vi "TCU Module (Main).vi"(7 "Name of Parent Panel":string="Main.vi", 9 "New Center Coords":T1={"Horizontal"=470, "Vertical"=200}, 10 "Config":variant, 11 "Main UI Message Queue":refnum<queue>) -> ()   [LabVIEW 2018, in "TCU Module.lvlib"]
doc: "This Continuous Measurement sample project is based on the Queued Message Handler template.\n\nThe Event Handling Loop generates messages based on user interface actions.\n\nThe Message Handling Loop processes messages generated by the Event Handling Loop, or by other messages. There are also Acquisition and Logging message handling loop subVIs, and a chart updating loop."
uses:
  TCU Module.lvlib
  support/Message Queue/Message Cluster.ctl
  <vilib>/Utility/miscctls.llb/LVPoint32TypeDef.ctl
  controls/UI Data.ctl
  controls/UI State.ctl
  TCU Module State Cluster.ctl
  TCU Module Config Cluster.ctl
  TCU Module Settings Cluster.ctl
  Measure Instrument/Output Devices.ctl
  Huber TCU/Huber Settings.ctl
  Lauda Integral XT-150 TCU/Lauda Settings.ctl
  Julabo Type 1 TCU/Julabo Type 1 TCU Folder/Julabo FP-50 Settings.ctl
  Huber Unistat 410 TCU/Huber Unistat 410 RS485 Settings.ctl
  Measure Instrument/State Enum.ctl
  Sequencing/Squence Update Cluster.ctl
  TCU Module Display.ctl
  support/Message Queue/Enqueue Message (Single).vi
  support/User Event - Stop/User Event - Stop.lvlib
  support/Support Library.lvlib
  support/Message Queue/Message Queue.lvlib
  Measure Instrument/TCU Module Engine.lvlib
  Measure Instrument/Feed Module Engine.lvlib
  Huber TCU/Huber Ministat 230 TCU.lvlib
  Lauda Integral XT-150 TCU/Lauda TCU.lvlib
  Julabo Type 1 TCU/Julabo Type 1 TCU Folder/Julabo Type FP-50 TCU.lvlib
  Sequencing/Sequencing Library.lvlib
  support/Command Log VIs/Command Logging.lvlib
  Huber Unistat 410 TCU/Huber Unistat 410 TCU.lvlib
  Report Generation/Report Generation.lvlib
panel:
  in  "Settings Button":bool
  out "Display Cluster":cluster{"User Name":string, "Temp Display":dbl}
  out "H/W":dbl
  out "Original Height":u32
  out "Original Width":u32
  out "TCU Image":u16(ring)
  out "TCU On?":bool
  out "ScanCode":i16
  out "Log File path":path
  out "Status":string
  in  "Exit":bool
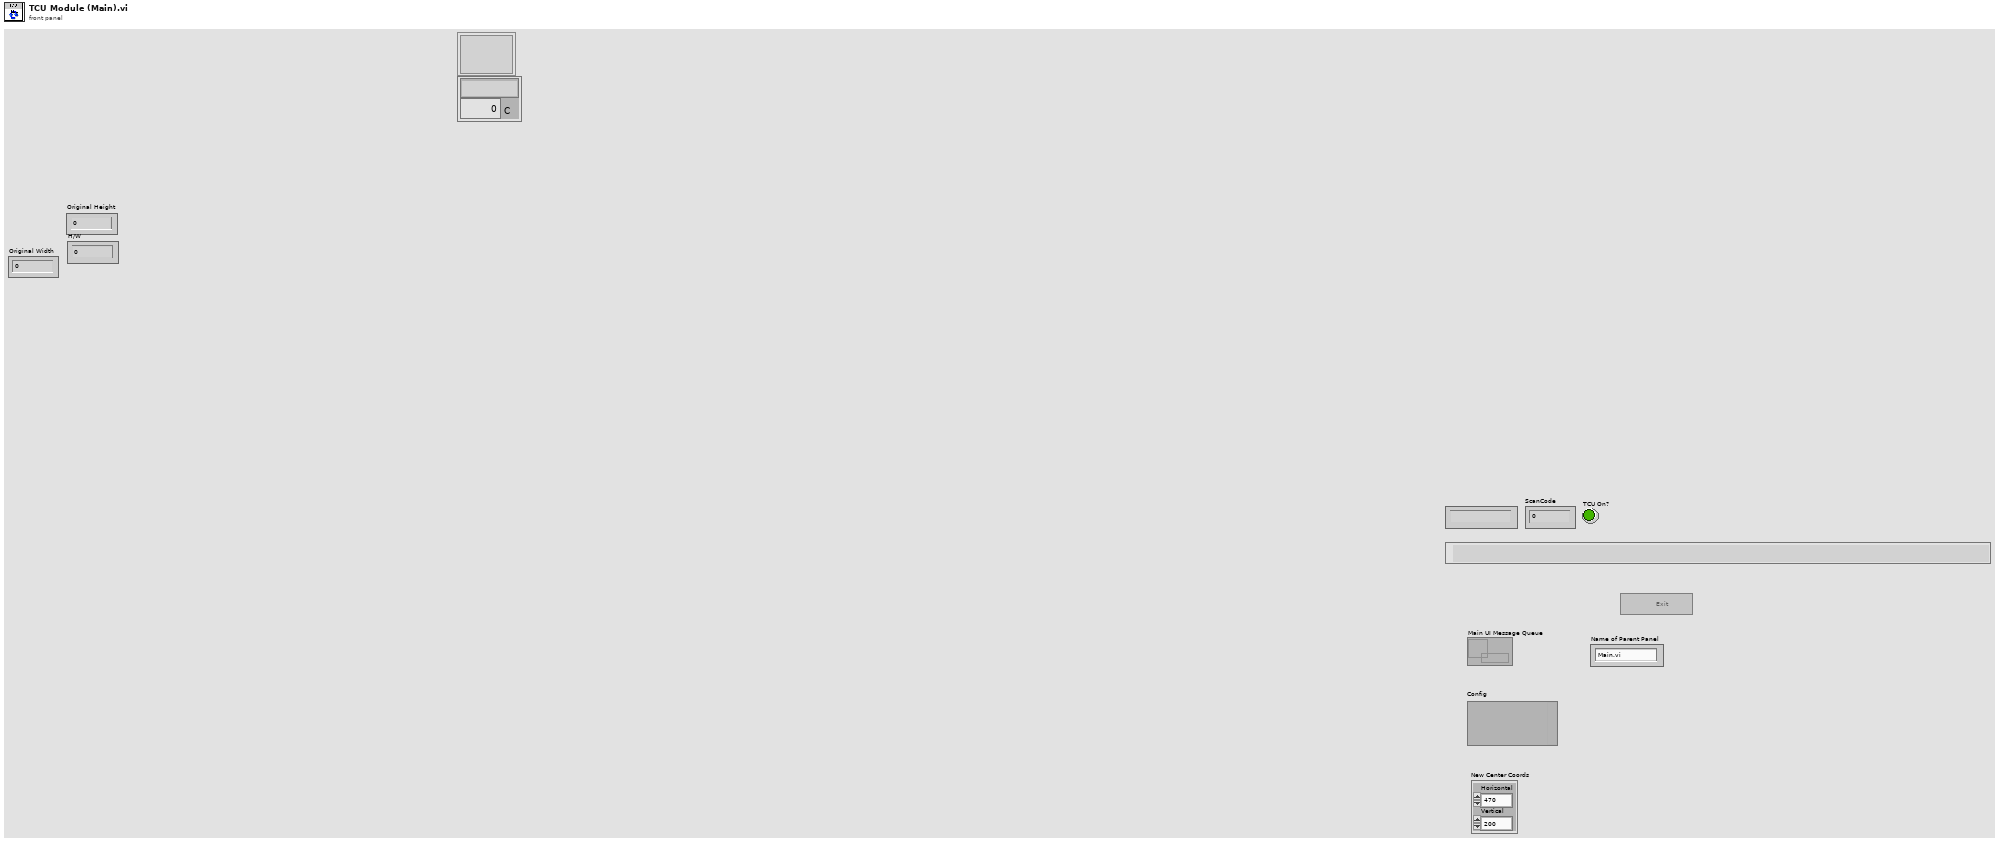
[diagram p1: front panel]
types:
  T1 = typedef "LVPoint32TypeDef.ctl" = cluster{"Horizontal":i32, "Vertical":i32}
  T2 = enum32{"Invalid", "Default", "Floating", "Floating/Auto-Hide", "Modal"}
  T3 = typedef "UI State.ctl" = enum16{"Idle", "Acquiring and Logging", "Waiting for Exit", "Waiting for Exit (Acq Stopped)", "Waiting for Exit (Log Stopped)", "Waiting for Stop", "Waiting for Stop (Acq Stopped)", "Waiting for Stop (Log Stopped)"}
  T4 = typedef "UI Data.ctl" = cluster{"Start Ref":refnum<vi>, "Trigger Ref":refnum<vi>, "Stop Ref":refnum<vi>, "Settings Ref":refnum<vi>, "Status Ref":refnum<vi>, "Exit Ref":refnum<vi>, "Data Ref":refnum<vi>}
  T5 = typedef "TCU Module.lvlib/TCU Module Config Cluster.ctl" = cluster{"GUID":string, "Drop Coords":T1, "Process Name":string, "User name":string, "Queue Name":string, "Settings":T6, "Load Count":i32, "Power Level Changed":bool}
  T6 = typedef "TCU Module.lvlib/TCU Module Settings Cluster.ctl" = cluster{"Cycle Period":dbl, "Setpoint Entry":dbl, "Output Device":T7, "Huber Ministat 230 Settings":T8, "Lauda Settings":T9, "Julabo FP-50 Settings":T10, "Internal Control?":bool, "Huber Unistat 410 Settings":T11}
  T7 = typedef "Output Devices.ctl" = enum16{"Default", "Huber Ministat 230", "Huber Unistat 410", "Lauda XT-150", "Julabo FP-50"}
  T8 = typedef "Huber Ministat 230 TCU.lvlib/Huber Settings.ctl" = cluster{"VISA resource name":refnum<visa-resource-name>, "Simulated?":bool}
  T9 = typedef "Lauda TCU.lvlib/Lauda Settings.ctl" = cluster{"VISA resource name":refnum<visa-resource-name>, "Simulated?":bool, "Pump Power":i32}
  T10 = typedef "Julabo Type FP-50 TCU.lvlib/Julabo FP-50 Settings.ctl" = cluster{"VISA resource name":refnum<visa-resource-name>, "Simulated?":bool, "Pump Power":i32}
  T11 = typedef "Huber Unistat 410 TCU.lvlib/Huber Unistat 410 RS485 Settings.ctl" = cluster{"VISA resource name":refnum<visa-resource-name>, "Address":i8, "Simulated?":bool}
  T12 = typedef "TCU Module.lvlib/TCU Module State Cluster.ctl" = cluster{"TCU Module Config":T5, "State":T13, "Start Time":timestamp, "Current Time":timestamp, "First Iteration":bool, "Data":cluster{"TCU Temp":dbl}, "Process Name":string, "TCU On?":bool, "Power Level Changed":bool}
  T13 = typedef "Feed Module.lvlib/Feed Module Engine.lvlib/State Enum.ctl" = enum16{"Measuring", "Idle", "Paused"}
  T14 = typedef "LVPointTypeDef.ctl" = cluster{"Horizontal":i16, "Vertical":i16}
  T15 = typedef "TCU Module.lvlib/All Message Queues.ctl" = cluster{"Engine":refnum<queue>, "TCU UI":refnum<queue>, "TCU Engine":refnum<queue>, "TCU Display":refnum<queue>}
  T16 = typedef "TCU Module.lvlib/TCU Module Display.ctl" = cluster{"TCU On?":bool, "Cycle Period":dbl, "Current TCU Temp":dbl}
  T17 = typedef "LVRectTypeDef.ctl" = cluster{"Left":i16, "Top":i16, "Right":i16, "Bottom":i16}
  T18 = cluster{"Shift":bool, "Ctrl":bool, "Alt":bool, "Cmd":bool, "Opt":bool}
  T19 = typedef "Sequencing Library.lvlib/Squence Update Cluster.ctl" = cluster{"Auto?":bool, "Manual Entry":dbl, "Setpoint":dbl}
  T20 = enum8{"Enabled", "Disabled", "Disabled and Grayed Out"}
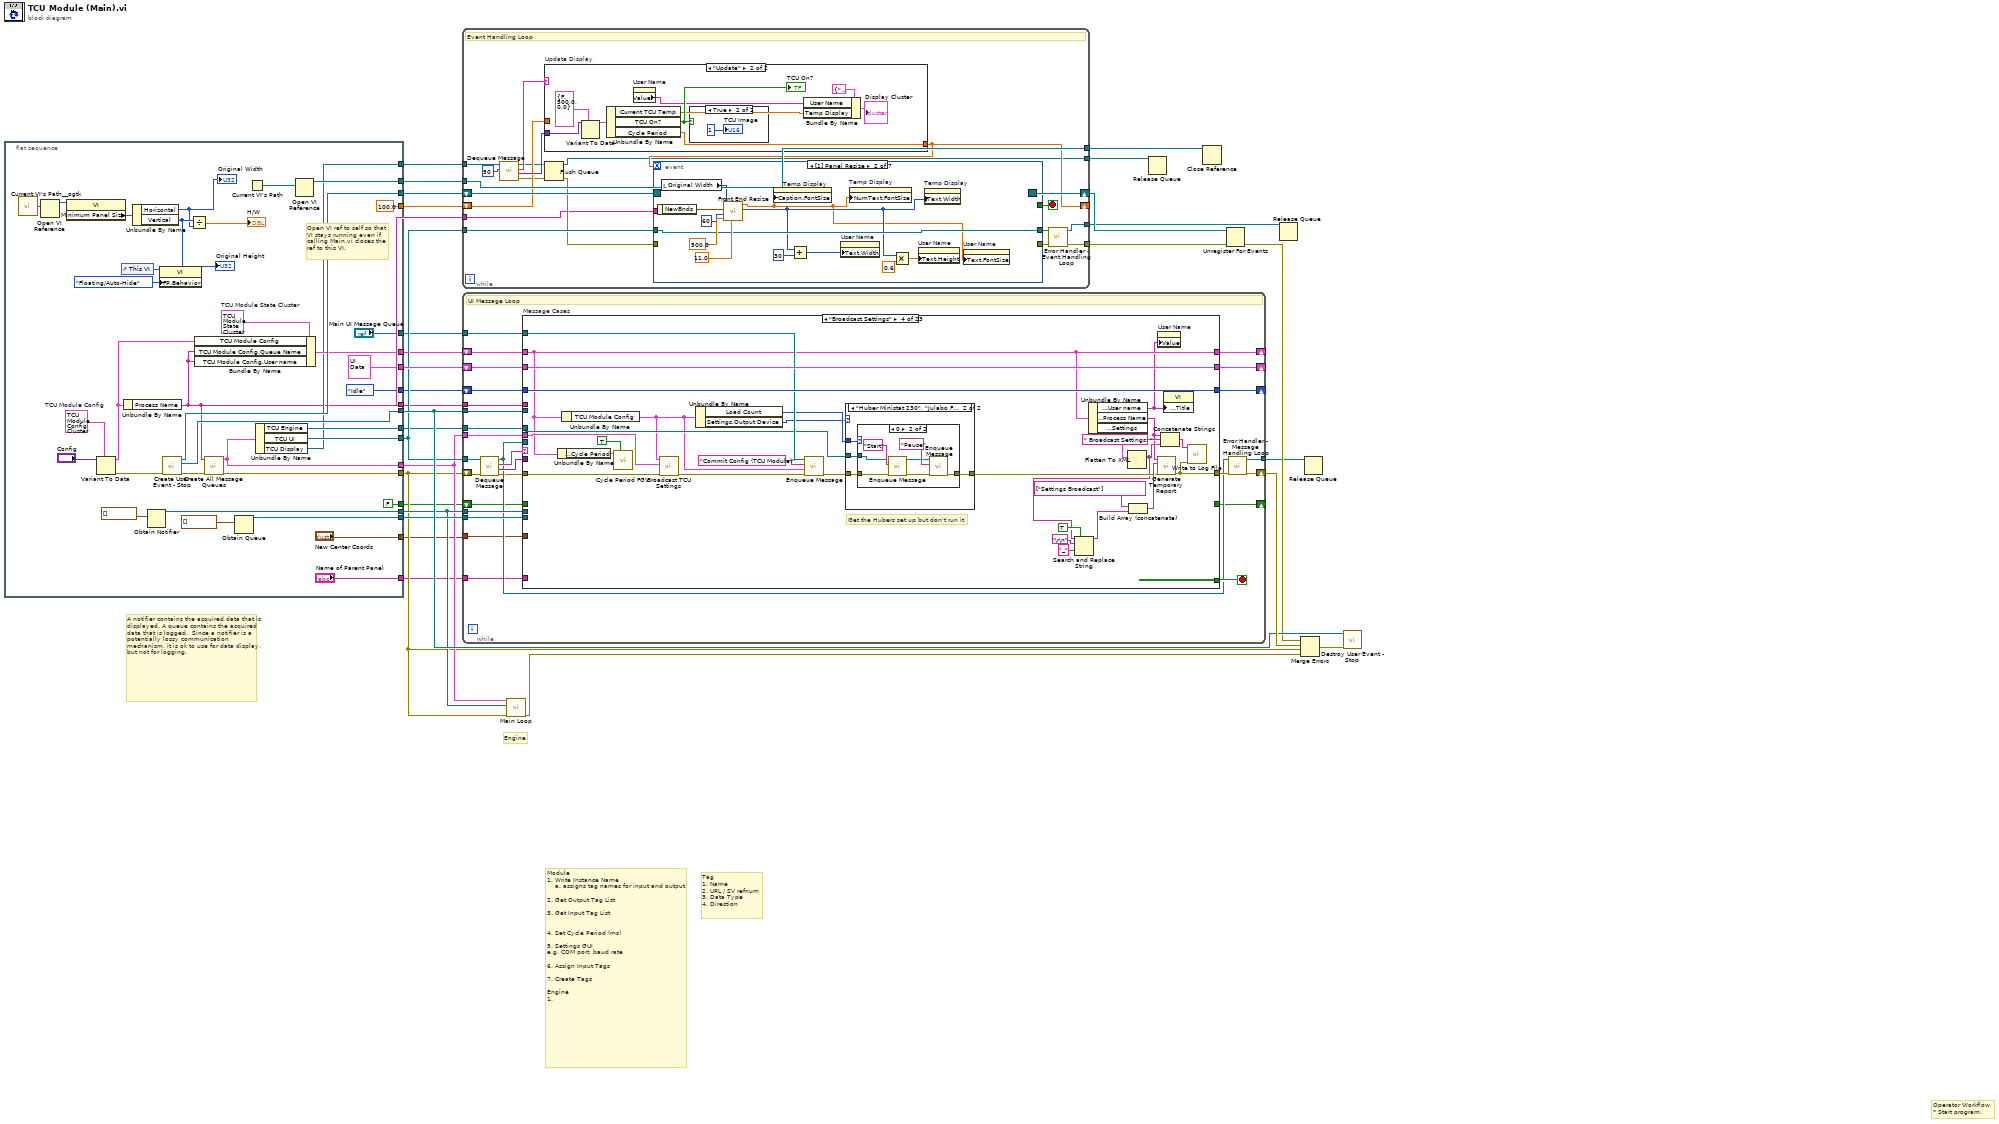
[diagram p0: block diagram]
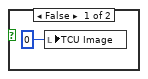
[diagram p3: hidden frame]
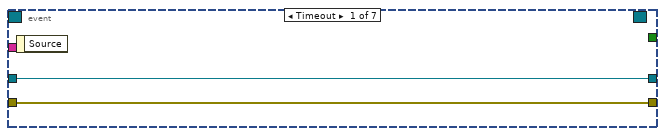
[diagram p4: hidden frame]
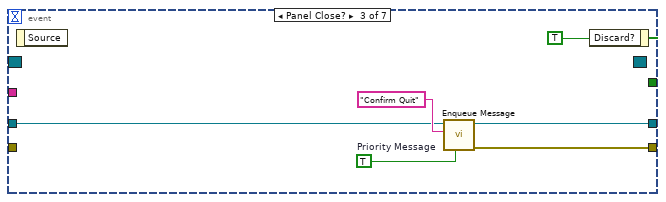
[diagram p5: hidden frame]
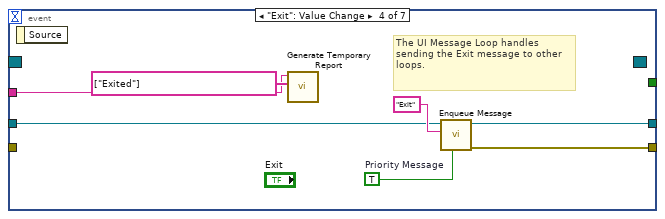
[diagram p6: hidden frame]
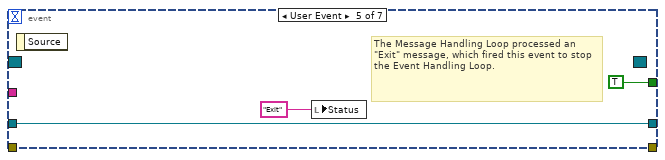
[diagram p7: hidden frame]
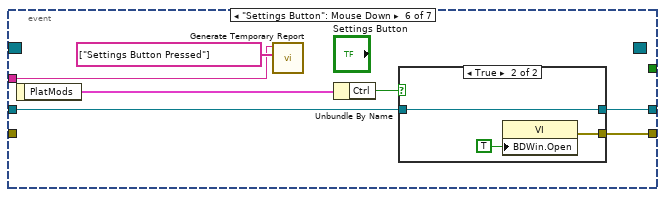
[diagram p8: hidden frame]
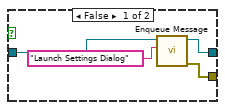
[diagram p9: hidden frame]
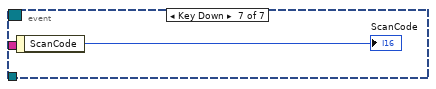
[diagram p10: hidden frame]
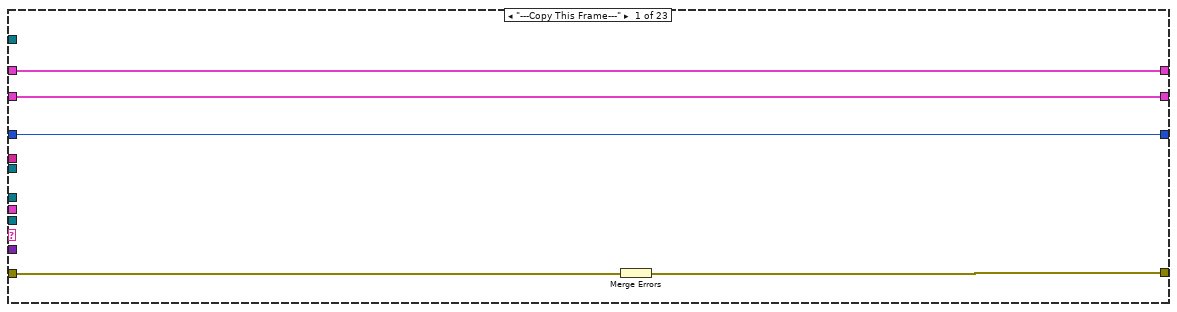
[diagram p11: hidden frame]
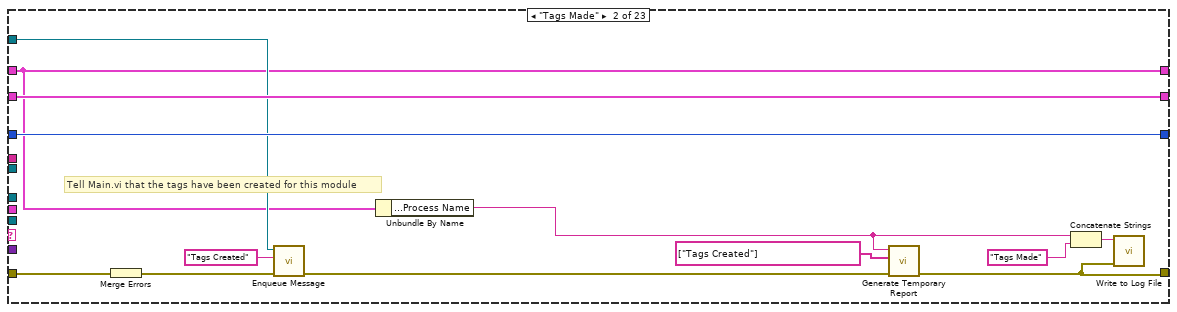
[diagram p12: hidden frame]
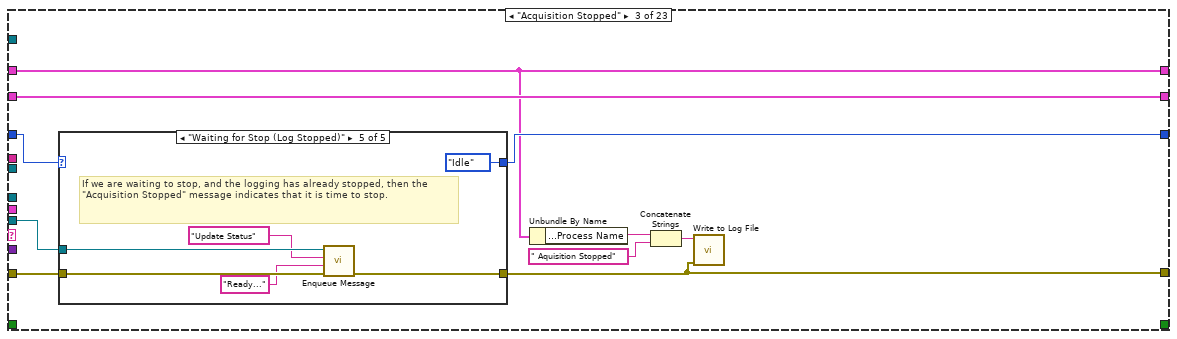
[diagram p13: hidden frame]
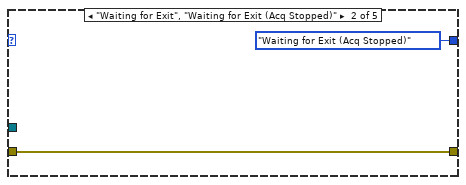
[diagram p15: hidden frame]
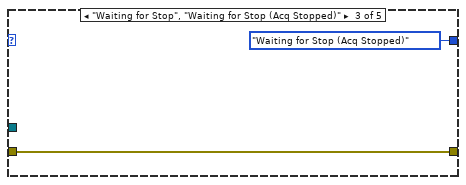
[diagram p16: hidden frame]
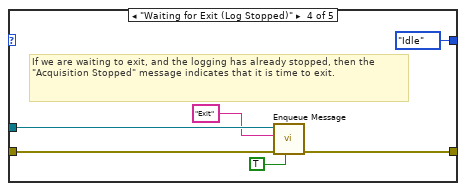
[diagram p17: hidden frame]
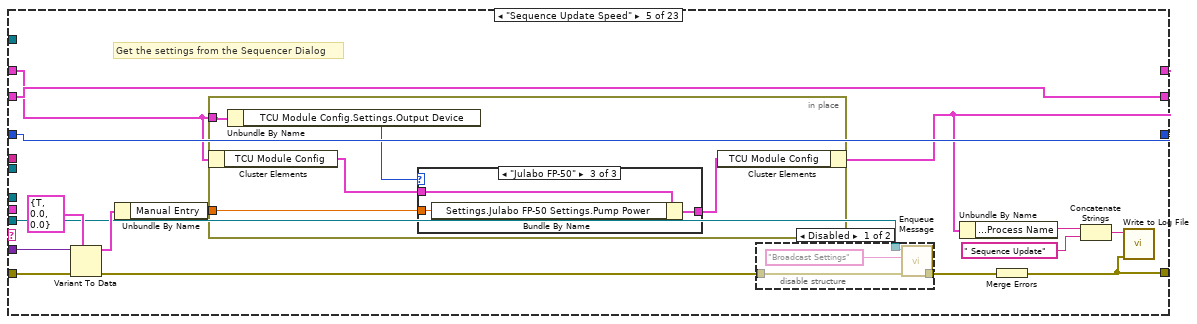
[diagram p20: hidden frame]
diagram:
  # "Engine"
  # "Operator Workflow\n* Start program."
  # "Module \n1. Write Instance Name\n    a. assigns tag names for input and output\n\n2. Get Output Tag List\n\n3. Get Input Tag List\n\n\n4. Set Cycle Period (ms)\n\n5. Settings GUI\ne.g. COM port, baud rate\n\n6. Assign Input Tags\n\n7. Create Tags\n\nEngine\n1."
  # "Tag\n1. Name\n2. URL / SV refnum\n3. Data Type\n4. Direction"
  # "A notifier contains the acquired data that is displayed. A queue contains the acquired data that is logged.  Since a notifier is a potentially lossy communication mechanism, it is ok to use for data display, but not for logging."
  n1 = flat-sequence {
    tunnel: [w65] -> w26
    tunnel: [w64] -> w25
    tunnel: [T4 {"Start Ref"=refnum, "Trigger Ref"=refnum, "Stop Ref"=refnum, "Settings Ref"=refnum, "Status Ref"=refnum, "Exit Ref"=refnum, "Data Ref"=refnum} ("Measurement UI Controls")] -> w22
    tunnel: [w62] -> w21
    tunnel: [UI_State."Idle" ("UI State")] -> w20
    tunnel: [w58] -> w19
    tunnel: [w57] -> w18
    tunnel: [w56] -> w16
    tunnel: [w55] -> w14
    tunnel: [w53] -> w13
    tunnel: ["Main UI Message Queue"] -> w12
    tunnel: [w48] -> w11
    tunnel: [w44] -> w10
    tunnel: [w43] -> w9
    tunnel: ["New Center Coords"] -> w8
    tunnel: ["Name of Parent Panel"] -> w7
    tunnel: [FALSE] -> w6
    tunnel: [100.0 ("Cycle Period")] -> w5
    tunnel: [w36] -> w1
    frame #0 {
      w46 = T5 {"GUID"="", "Drop Coords"={"Horizontal"=0, "Vertical"=0}, "Process Name"="", "User name"="", "Queue Name"="", "Settings"={"Cycle Period"=500.0, "Setpoint Entry"=0.0, "Output Device"=enum."Default", "Huber Ministat 230 Settings"={"VISA resource name"="", "Simulated?"=TRUE}, "Lauda Settings"={"VISA resource name"="", "Simulated?"=FALSE, "Pump Power"=2}, "Julabo FP-50 Settings"={"VISA resource name"="", "Simulated?"=FALSE, "Pump Power"=2}, "Internal Control?"=FALSE, "Huber Unistat 410 Settings"={"VISA resource name"="", "Address"=0, "Simulated?"=FALSE}}, "Load Count"=0, "Power Level Changed"=FALSE}  # TCU Module Config
      w49 = T12 {"TCU Module Config"={"GUID"="", "Drop Coords"={"Horizontal"=0, "Vertical"=0}, "Process Name"="", "User name"="", "Queue Name"="", "Settings"={"Cycle Period"=500.0, "Setpoint Entry"=0.0, "Output Device"=enum."Default", "Huber Ministat 230 Settings"={"VISA resource name"="", "Simulated?"=TRUE}, "Lauda Settings"={"VISA resource name"="", "Simulated?"=FALSE, "Pump Power"=2}, "Julabo FP-50 Settings"={"VISA resource name"="", "Simulated?"=FALSE, "Pump Power"=2}, "Internal Control?"=FALSE, "Huber Unistat 410 Settings"={"VISA resource name"="", "Address"=0, "Simulated?"=FALSE}}, "Load Count"=0, "Power Level Changed"=FALSE}, "State"=enum."Idle", "Start Time"=timestamp(0 s since 1904-01-01), "Current Time"=timestamp(0 s since 1904-01-01), "First Iteration"=FALSE, "Data"={"TCU Temp"=0.0}, "Process Name"="", "TCU On?"=FALSE, "Power Level Changed"=FALSE}  # TCU Module State Cluster
      # "Open VI ref to self so that\nVI stays running even if\ncalling Main.vi closes the\nref to this VI."
      n2 = call <userlib>:"Current VI's Path__ogtk.vi"() -> ("Current VI's Path (+ Relative)"=w31:path)  [unwired: 1 in]
      n3 = Open VI Reference(vi path=w31) -> (vi reference=w32:refnum<vi>)  [unwired: 5 in, 1 out]
      n4 = property class="VI"(reference=w32) -> ("Minimum Panel Size"=w33:T14)  [unwired: 1 in, 2 out]
      n5 = Variant To Data(type=w46, Variant="Config") -> (data=w51:T5, error out=w52:errorcluster)  [unwired: 1 in]
      n6 = control-ref of="This VI"() -> (w38:refnum<vi>)
      n7 = Unbundle By Name(w51) -> ("Process Name"=w36:string)
      n8 = Unbundle By Name(w33) -> ("Horizontal"=w34:i16, "Vertical"=w35:i16)
      "Original Width" <- w34
      "Original Height" <- w35
      n9 = Obtain Notifier(notification data type=waveform(dbl)[] []) -> (notifier out=w56:refnum<notifier>)  [unwired: 3 in, 2 out]
      n10 = property class="VI"(reference=w38, "FP.Behavior"=T2."Floating/Auto-Hide" ("Front Panel Window:Behavior")) -> ()  [unwired: 1 in, 2 out]
      n11 = call "Create User Event - Stop.vi"("error in (no error)"=w52) -> ("error out"=w45:errorcluster, "User Event - Stop"=w64:refnum<user-event>, "Stop Event Registration Refnum"=w65:refnum<event-registration>)  [unwired: 8 in]
      n12 = Divide(x=w35, y=w34) -> (x/y=→"H/W":dbl)
      n13 = Bundle By Name(cluster=w49, "TCU Module Config"=w51, "TCU Module Config.Queue Name"=w36, "TCU Module Config.User name"=w36) -> (w53:T12)
      n14 = call "Create All Message Queues.vi"("error in (no error)"=w45, "Process Name"=w36) -> ("error out"=w43:errorcluster, "Message Queues"=w44:T15)  [unwired: 8 in]
      n15 = Obtain Queue(element data type=waveform(dbl)[] []) -> (queue out=w57:refnum<queue>)  [unwired: 4 in, 2 out]
      n16 = Current VI's Path() -> (path=w54:path)
      n17 = Unbundle By Name(w44) -> ("TCU Engine"=w58:refnum<queue>, "TCU UI"=w62:refnum<queue>, "TCU Display"=w48:refnum<queue>)
      n18 = Open VI Reference(vi path=w54) -> (vi reference=w55:refnum<vi>)  [unwired: 5 in, 1 out]
    }
  }
  n19 = while {
    tunnel: w21 -> [w79]
    tunnel: [w81] -> w28
    shift-right: [w80] -> w23
    shift-left: w26 -> [w85]
    tunnel: [w78] -> w15
    tunnel: w14 -> [w78]
    tunnel: w11 -> [w77]
    shift-right: [w74] -> _
    shift-left: w5 -> [w73]
    tunnel: [w69] -> w3
    tunnel: [w68] -> w4
    tunnel: w1 -> [w66]
    stop <- w84 stop-if-true
    # "Event Handling Loop"
    n20 = call "Dequeue Message.vi"("timeout in ms (-1)"=50, "Message Queue"=w77) -> ("error out"=w70:errorcluster, "Message Data"=w75:variant, "Message"=w76:string, "dup Message Queue"=w71:refnum<queue>)  [unwired: 6 in]
    n21 = case "Update Display" shown="\"Update\"" w76 {
      tunnel: w75 -> [_ w95]
      tunnel: [w86 w92] -> w74
      tunnel: w73 -> [w86 _]
      frame "False", Default {
      }
      frame "Update" {
        n22 = Variant To Data(type=T16 {"TCU On?"=FALSE, "Cycle Period"=500.0, "Current TCU Temp"=0.0} ("FM Display"), Variant=w95) -> (data=w94:T16)  [unwired: 1 in, 1 out]
        n23 = Unbundle By Name(w94) -> ("Current TCU Temp"=w90:dbl, "TCU On?"=w93:bool, "Cycle Period"=w92:dbl)
        "TCU On?" <- w93
        n24 = property on="User Name" class="Str"() -> ("Value"=w87:string)  [unwired: 2 in, 2 out]
        n25 = case shown="True" w93 {
          frame False {
            n26 = local write "TCU Image"(u16 0 ("Ring")) -> ()
          }
          frame True {
            "TCU Image" <- u16 1 ("Ring")
          }
        }
        n27 = Bundle By Name(cluster=cluster{"User Name":string, "Temp Display":dbl} {"User Name"="", "Temp Display"=0.0} ("Display Cluster"), "User Name"=w87, "Temp Display"=w90) -> (→"Display Cluster":cluster{"User Name":string, "Temp Display":dbl})
      }
    }
    n28 = Flush Queue(queue=w71, error in (no error)=w70) -> (queue out=w68:refnum<queue>, error out=w67:errorcluster)  [unwired: 1 out]
    n29 = event shown="[1] Panel Resize" {
      selector: w85 -> [_ _ _ _ _ _ _]
      dyn-events: [_ _ _ _ _ _ _] -> w80
      timeout: w74 -> [_ _ _ _ _ _ _]
      tunnel: [_ _ _ _ TRUE ("Discard?") _ _] -> w84
      tunnel: w79 -> [w99 w106 w114 w121 w125 w132 _]
      tunnel: [w98 _ w112 w124 _ w134 _] -> w82
      tunnel: [w99 w106 w113 w120 w125 w133 _] -> w83
      tunnel: w67 -> [w98 _ _ _ _ _ _]
      tunnel: w66 -> [_ _ _ w118 _ w128 _]
      event Timeout {
        n30 = event-data() -> ()  [unwired: 1 in, 1 out]
      }
      event Panel Resize {
        n31 = event-data() -> ("NewBnds"=w108:T17)  [unwired: 1 in]
        n32 = local read "Original Width"() -> (w107:u32)
        n33 = call "Front End Resize.vi"("Starting Font"=11.0, "Area to Font Division"=500.0, "Original Text Box Width"=60, "NewBnds"=w108, "Original Panel Width"=w107) -> ("New Text Box Width"=w101:u64, "New Font Size"=w100:dbl)  [unwired: 5 in]
        n34 = property on="Temp Display" class="DigNum (strict)"("Caption.FontSize"=w100) -> ()  [unwired: 2 in, 2 out]
        n35 = Add(x=w101, y=u64 30) -> (x+y=w102:u64)
        n36 = property on="User Name" class="Str"("Text.Width"=w102) -> ()  [unwired: 2 in, 2 out]
        n37 = property on="Temp Display" class="DigNum (strict)"("NumText.FontSize"=w100) -> ()  [unwired: 2 in, 2 out]
        n38 = Multiply(x=w101, y=0.6) -> (x*y=w105:dbl)
        n39 = property on="User Name" class="Str"("Text.Height"=w105) -> ()  [unwired: 2 in, 2 out]
        n40 = property on="Temp Display" class="DigNum (strict)"("Text Width"=w101) -> ()  [unwired: 2 in, 2 out]
        n41 = property on="User Name" class="Str"("Text.FontSize"=w100) -> ()  [unwired: 2 in, 2 out]
      }
      event Panel Close? {
        w115 = TRUE  # Priority Message
        n42 = event-data() -> ()  [unwired: 1 in, 1 out]
        n43 = call-poly "Enqueue Message.vi"("Priority Message? (F)"=w115, "Message"="Confirm Quit", "Message Queue"=w114) -> ("error out"=w112:errorcluster, "dup Message Queue"=w113:refnum<queue>)  [unwired: 7 in]
        n44 = event-data("Discard?"=TRUE) -> ()  [unwired: 1 in, 1 out]
      }
      event "Exit": Value Change {
        w122 = TRUE  # Priority Message
        # "The UI Message Loop handles sending the Exit message to other loops."
        n45 = event-data() -> ()  [unwired: 1 in, 1 out]
        n46 = call "Generate Temporary Report.vi"("Line of Events"=string[] ["Exited"], "Module Name"=w118) -> ()  [unwired: 9 in, 1 out]
        n47 = call-poly "Enqueue Message.vi"("Priority Message? (F)"=w122, "Message"="Exit", "Message Queue"=w121) -> ("error out"=w124:errorcluster, "dup Message Queue"=w120:refnum<queue>)  [unwired: 7 in]
      }
      event User Event {
        # "The Message Handling Loop processed an \"Exit\" message, which fired this event to stop the Event Handling Loop."
        n48 = event-data() -> ()  [unwired: 1 in, 1 out]
        n49 = local write "Status"("Exit" ("Exit String")) -> ()
      }
      event "Settings Button": Mouse Down {
        n50 = event-data() -> ("PlatMods"=w131:T18)  [unwired: 1 in]
        n51 = call "Generate Temporary Report.vi"("Line of Events"=string[] ["Settings Button Pressed"], "Module Name"=w128) -> ()  [unwired: 9 in, 1 out]
        n52 = Unbundle By Name(w131) -> ("Ctrl"=w130:bool)
        n53 = case shown="True" w130 {
          tunnel: [w138 w139] -> w134
          tunnel: [w137 w140] -> w133
          tunnel: w132 -> [w136 w140]
          frame False {
            n54 = call-poly "Enqueue Message.vi"("Message"="Launch Settings Dialog", "Message Queue"=w136) -> ("error out"=w138:errorcluster, "dup Message Queue"=w137:refnum<queue>)  [unwired: 8 in]
          }
          frame True {
            n55 = property class="VI"("BDWin.Open"=TRUE ("Block Diagram Window:Open")) -> (error out=w139:errorcluster)  [unwired: 2 in, 1 out]
          }
        }
      }
      event Key Down {
        n56 = event-data() -> ("ScanCode"=→"ScanCode":i16)  [unwired: 1 in]
      }
    }
    n57 = call "Error Handler - Event Handling Loop.vi"("error in (no error)"=w82, "Message Queue"=w83) -> ("dup error in"=w81:errorcluster, "dup Message Queue"=w69:refnum<queue>)  [unwired: 8 in]
  }
  n58 = while {
    tunnel: w21 -> [w164]
    tunnel: w25 -> [w168]
    shift-right: [w158] -> w29
    shift-left: w9 -> [w167]
    shift-right: [w150] -> _
    shift-left: w13 -> [w152]
    shift-right: [w162] -> _
    shift-left: w22 -> [w163]
    tunnel: w16 -> [w161]
    tunnel: w18 -> [w160]
    shift-right: [w155] -> _
    shift-left: w20 -> [w156]
    tunnel: w19 -> [w154]
    tunnel: w12 -> [w151]
    tunnel: w10 -> [w149]
    tunnel: w1 -> [w148]
    tunnel: w8 -> [w147]
    tunnel: w7 -> [w146]
    shift-right: [w145] -> _
    shift-left: w6 -> [w144]
    tunnel: [w143] -> w2
    stop <- w169 stop-if-true
    # "UI Message Loop"
    n59 = call "Dequeue Message.vi"("error in (no error)"=w167, "Message Queue"=w164) -> ("error out"=w153:errorcluster, "Message Data"=w165:variant, "Message"=w166:string, "dup Message Queue"=w157:refnum<queue>)  [unwired: 6 in]
    n60 = case "Message Cases" shown="\"Broadcast Settings\"" w166 {
      selector: w166 -> [_ _ _ _ _ _ _ _ _ _ _ _ _ _ _ _ _ _ _ _ _ _ w692]
      tunnel: w157 -> [_ _ w193 _ w266 w298 w317 _ w386 w400 w427 _ w467 w487 w510 _ w557 w588 _ _ w647 _ _]
      tunnel: w153 -> [w174 w187 w194 w240 w265 w297 w316 w352 w367 w404 w431 w450 w462 w485 w511 w538 w555 w587 w611 w623 w645 w684 _]
      tunnel: [w173 w175 w190 w220 w260 w292 w314 w353 w358 w391 w406 w450 w451 w479 w506 w542 w546 w573 w607 w625 w640 w685 w691] -> w159
      tunnel: [_ _ _ _ _ _ _ _ _ _ TRUE _ _ _ _ _ _ _ _ _ _ _ _] -> w169
      tunnel: w165 -> [_ _ _ _ w264 w296 _ w355 _ w403 w413 _ _ _ _ w535 _ _ _ _ _ w683 _]
      tunnel: w168 -> [_ _ _ _ _ _ _ _ _ _ w430 _ _ _ _ _ _ _ _ _ _ _ _]
      tunnel: w152 -> [w170 w179 w189 w228 w259 w291 w313 w350 w365 w390 w410 w441 w455 w476 w505 w540 w551 w583 w612 w624 w653 w674 w697]
      tunnel: w163 -> [w172 w186 w197 w244 w268 w300 w319 w357 w383 w405 w428 w449 w463 w490 w514 w544 w552 w584 w617 w634 w669 w680 w702]
      tunnel: [w172 w186 w197 w244 w268 w300 w319 w357 w383 w405 w428 w448 w463 w490 w514 w544 w552 w584 w617 w634 w669 w680 w702] -> w162
      tunnel: w161 -> [_ _ _ _ _ _ _ _ _ _ w426 _ _ _ _ _ _ _ _ _ _ _ _]
      tunnel: w160 -> [_ _ _ _ _ _ _ _ _ _ w422 _ _ _ _ _ _ _ _ _ _ _ _]
      tunnel: w156 -> [w171 w185 w196 w243 w267 w299 w318 w351 w372 w395 _ _ _ w489 w513 w541 _ _ _ _ w658 w675 w701]
      tunnel: [w171 w185 w195 w243 w267 w299 w315 w351 w373 w395 UI_State."Idle" ("UI State") UI_State."Idle" ("UI State") UI_State."Idle" ("UI State") w489 w512 w541 UI_State."Acquiring and Logging" ("UI State") UI_State."Acquiring and Logging" ("UI State") UI_State."Acquiring and Logging" ("UI State") UI_State."Acquiring and Logging" ("UI State") w659 w675 w701] -> w155
      tunnel: w154 -> [_ _ _ w233 _ _ _ _ w371 _ w420 _ _ _ _ _ _ _ w615 w632 w657 _ _]
      tunnel: w151 -> [_ w183 _ w239 _ _ _ _ _ _ w414 _ _ w488 _ _ _ _ _ _ _ _ _]
      tunnel: [w170 w179 w189 w228 w258 w290 w313 w350 w362 w390 w410 w441 w455 w478 w505 w540 w545 w572 w612 w624 w649 w674 w697] -> w150
      tunnel: w149 -> [_ _ _ w236 _ _ _ _ _ _ _ _ _ w483 _ _ _ _ _ _ _ _ _]
      tunnel: w148 -> [_ _ _ _ _ _ _ _ _ _ _ _ w458 _ _ _ _ _ _ _ _ _ _]
      tunnel: w147 -> [_ _ _ _ _ _ _ _ _ _ _ _ w460 _ _ _ _ _ _ _ _ _ _]
      tunnel: w146 -> [_ _ _ _ _ _ _ _ _ _ _ _ w459 _ _ _ _ _ _ _ _ _ _]
      tunnel: w144 -> [_ _ _ _ _ _ _ _ _ _ _ _ _ _ _ _ _ w578 _ _ _ _ _]
      tunnel: [_ _ _ _ _ _ _ _ _ _ _ _ _ _ _ _ _ w577 _ _ _ _ _] -> w145
      frame "---Copy This Frame---" {
        # "Duplicate this frame when creating new messages.  Change this comment in the duplicated frame to describe this message."
        n61 = Merge Errors(w174) -> (w173:errorcluster)
      }
      frame "Tags Made" {
        # "Tell Main.vi that the tags have been created for this module"
        # "Duplicate this frame when creating new messages.  Change this comment in the duplicated frame to describe this message."
        n62 = Merge Errors(w187) -> (w182:errorcluster)
        n63 = call-poly "Enqueue Message.vi"("error in (no error)"=w182, "Message"="Tags Created", "Message Queue"=w183) -> ("error out"=w176:errorcluster)  [unwired: 7 in, 1 out]
        n64 = Unbundle By Name(w179) -> ("TCU Module Config.Process Name"=w177:string)
        n65 = call "Generate Temporary Report.vi"("error in (no error)"=w176, "Line of Events"=string[] ["Tags Created"], "Module Name"=w177) -> ("error out"=w175:errorcluster)  [unwired: 8 in]
        n66 = Concatenate Strings(w177, "Tags Made" ("text")) -> (w180:string)
        n67 = call "Write to Log File.vi"("error in"=w175, "text"=w180) -> ()  [unwired: 9 in, 1 out]
      }
      frame "Acquisition Stopped" {
        # "Logic for determining what action to take when the acquisition has stopped."
        n68 = case shown="\"Waiting for Stop (Log Stopped)\"" w196 {
          selector: w196 -> [w199 _ _ _ _]
          tunnel: [w199 UI_State."Waiting for Exit (Acq Stopped)" ("UI State") UI_State."Waiting for Stop (Acq Stopped)" ("UI State") UI_State."Idle" ("UI State") UI_State."Idle" ("UI State")] -> w195
          tunnel: w194 -> [w198 w200 w202 w208 w214]
          tunnel: [w198 w200 w202 w207 w213] -> w190
          tunnel: w193 -> [_ _ _ w206 w212]
          frame Default {
          }
          frame "Waiting for Exit", "Waiting for Exit (Acq Stopped)" {
          }
          frame "Waiting for Stop", "Waiting for Stop (Acq Stopped)" {
          }
          frame "Waiting for Exit (Log Stopped)" {
            # "If we are waiting to exit, and the logging has already stopped, then the \"Acquisition Stopped\" message indicates that it is time to exit."
            n69 = call-poly "Enqueue Message.vi"("Priority Message? (F)"=TRUE, "error in (no error)"=w208, "Message"="Exit", "Message Queue"=w206) -> ("error out"=w207:errorcluster)  [unwired: 6 in, 1 out]
          }
          frame "Waiting for Stop (Log Stopped)" {
            # "If we are waiting to stop, and the logging has already stopped, then the \"Acquisition Stopped\" message indicates that it is time to stop."
            n70 = call-poly "Enqueue Message.vi"("error in (no error)"=w214, "Message Data"="Ready..." ("Message"), "Message"="Update Status", "Message Queue"=w212) -> ("error out"=w213:errorcluster)  [unwired: 6 in, 1 out]
          }
        }
        n71 = Unbundle By Name(w189) -> ("TCU Module Config.Process Name"=w192:string)
        n72 = Concatenate Strings(w192, " Aquisition Stopped" ("text")) -> (w191:string)
        n73 = call "Write to Log File.vi"("error in"=w190, "text"=w191) -> ()  [unwired: 9 in, 1 out]
      }
      frame "Broadcast Settings" {
        # "Get the Hubers set up but don't run it"
        # "Send the 'Update Settings' message to the Logging and Acquisition message loops."
        n74 = Unbundle By Name(w228) -> ("TCU Module Config.Settings.Cycle Period"=w241:dbl)
        n75 = Unbundle By Name(w228) -> ("TCU Module Config"=w231:T5)
        n76 = call "Cycle Period FGV.vi"("Write"=TRUE, "Cycle Period In (ms)"=w241) -> ()  [unwired: 8 in, 2 out]
        n77 = call "Broadcast TCU Settings.vi"("error in (no error)"=w240, "Message Queues"=w236, "Pump Module Config"=w231) -> ("error out"=w238:errorcluster)  [unwired: 8 in]
        n78 = Unbundle By Name(w231) -> ("Load Count"=w235:i32, "Settings.Output Device"=w232:T7)
        n79 = call-poly "Enqueue Message.vi"("error in (no error)"=w238, "Message Data"=w231, "Message"="Commit Config (TCU Module)", "Message Queue"=w239) -> ("error out"=w234:errorcluster)  [unwired: 6 in, 1 out]
        n80 = case shown="\"Huber Ministat 230\", \"Julabo FP-50\"" w232 {
          tunnel: w234 -> [w245 w249]
          tunnel: w233 -> [_ w248]
          tunnel: [w245 w247] -> w221
          tunnel: w235 -> [_ w246]
          frame "Default", Default {
          }
          frame "Huber Ministat 230", "Julabo FP-50" {
            n81 = case shown="0" w246 {
              tunnel: w249 -> [w250 w254]
              tunnel: w248 -> [_ w253]
              tunnel: [w250 w257] -> w247
              frame Default {
              }
              frame 0 {
                n82 = call-poly "Enqueue Message.vi"("error in (no error)"=w254, "Message"="Start", "Message Queue"=w253) -> ("error out"=w251:errorcluster, "dup Message Queue"=w252:refnum<queue>)  [unwired: 7 in]
                n83 = call-poly "Enqueue Message.vi"("error in (no error)"=w251, "Message"="Pause", "Message Queue"=w252) -> ("error out"=w257:errorcluster)  [unwired: 7 in, 1 out]
              }
            }
          }
        }
        n84 = Unbundle By Name(w228) -> ("TCU Module Config.User name"=w216:string, "TCU Module Config.Process Name"=w219:string, "TCU Module Config.Settings"=w227:T6)
        n85 = Flatten To XML(anything=w227) -> (xml string=w218:string)
        n86 = Search and Replace String(replace all?=TRUE ("replace all? (F)"), input string=w218, search string="\r\n", replace string="_" ("replace string (\"\")")) -> (result string=w217:string)  [unwired: 4 in, 3 out]
        n87 = Build Array (concatenate)(string[] ["Settings Broadcast"] ("Line of Events"), w217) -> (w222:string[])
        n88 = call "Generate Temporary Report.vi"("error in (no error)"=w221, "Line of Events"=w222, "Module Name"=w219) -> ("error out"=w220:errorcluster)  [unwired: 8 in]
        n89 = property on="User Name" class="Str"("Value"=w216) -> ()  [unwired: 2 in, 2 out]
        n90 = Concatenate Strings(w219, " Broadcast Settings: " ("text"), w218) -> (w230:string)
        n91 = property class="VI"("Front Panel.Title"=w216) -> ()  [unwired: 2 in, 2 out]
        n92 = call "Write to Log File.vi"("error in"=w220, "text"=w230) -> ()  [unwired: 9 in, 1 out]
      }
      frame "Sequence Update Speed" {
        # "Get the settings from the Sequencer Dialog"
        # "Send the 'Update Settings' message to the Logging and Acquisition message loops."
        n93 = Variant To Data(error in=w265, type=T19 {"Auto?"=TRUE, "Manual Entry"=0.0, "Setpoint"=0.0} ("Cluster"), Variant=w264) -> (data=w272:T19, error out=w269:errorcluster)
        n94 = Unbundle By Name(w272) -> ("Manual Entry"=w271:dbl)
        n95 = in-place {
          in-place-border: w271 -> [w282]
          in-place-border: w259 -> [w281]
          n96 = in-place-cluster #1(w259) -> ("TCU Module Config"=w279:T5)
          n97 = Unbundle By Name(w281) -> ("TCU Module Config.Settings.Output Device"=w280:T7)
          n98 = case shown="\"Julabo FP-50\"" w280 {
            tunnel: w279 -> [w283 w286 w289]
            tunnel: w282 -> [_ w285 w288]
            tunnel: [w283 w284 w287] -> w278
            frame "Default", Default {
            }
            frame "Lauda XT-150" {
              n99 = Bundle By Name(cluster=w286, "Settings.Lauda Settings.Pump Power"=w285) -> (w284:T5)
            }
            frame "Julabo FP-50" {
              n100 = Bundle By Name(cluster=w289, "Settings.Julabo FP-50 Settings.Pump Power"=w288) -> (w287:T5)
            }
          }
          n101 = in-place-cluster #1("TCU Module Config"=w278) -> (w258:T12)
        }
        n102 = disable-structure shown="Disabled" {
          disable-tunnel: [w277 _] -> w270
          disable-tunnel: w269 -> [w275 _]
          disable-tunnel: w266 -> [w274 _]
          frame Disabled {
            n103 = call-poly "Enqueue Message.vi"("error in (no error)"=w275, "Message"="Broadcast Settings", "Message Queue"=w274) -> ("error out"=w277:errorcluster)  [unwired: 7 in, 1 out]
          }
          frame Enabled {
          }
        }
        n104 = Unbundle By Name(w258) -> ("TCU Module Config.Process Name"=w263:string)
        n105 = Merge Errors(w270) -> (w260:errorcluster)
        n106 = Concatenate Strings(w263, " Sequence Update" ("text")) -> (w262:string)
        n107 = call "Write to Log File.vi"("error in"=w260, "text"=w262) -> ()  [unwired: 9 in, 1 out]
      }
      frame "Sequence Update Temperature" {
        # "Get the settings from the Sequencer Dialog"
        # "Send the 'Update Settings' message to the Logging and Acquisition message loops."
        n108 = Variant To Data(error in=w297, type=T19 {"Auto?"=TRUE, "Manual Entry"=0.0, "Setpoint"=0.0} ("Cluster"), Variant=w296) -> (data=w304:T19, error out=w301:errorcluster)
        n109 = Unbundle By Name(w304) -> ("Manual Entry"=w303:dbl)
        n110 = in-place {
          in-place-border: w303 -> [w312]
          n111 = in-place-cluster #2(w291) -> ("TCU Module Config"=w310:T5)
          n112 = Bundle By Name(cluster=w310, "Settings.Setpoint Entry"=w312) -> (w311:T5)
          n113 = in-place-cluster #2("TCU Module Config"=w311) -> (w290:T12)
        }
        n114 = disable-structure shown="Disabled" {
          disable-tunnel: [w309 _] -> w302
          disable-tunnel: w301 -> [w307 _]
          disable-tunnel: w298 -> [w306 _]
          frame Disabled {
            n115 = call-poly "Enqueue Message.vi"("error in (no error)"=w307, "Message"="Broadcast Settings", "Message Queue"=w306) -> ("error out"=w309:errorcluster)  [unwired: 7 in, 1 out]
          }
          frame Enabled {
          }
        }
        n116 = Unbundle By Name(w290) -> ("TCU Module Config.Process Name"=w295:string)
        n117 = Merge Errors(w302) -> (w292:errorcluster)
        n118 = Concatenate Strings(w295, " Sequence Update" ("text")) -> (w294:string)
        n119 = call "Write to Log File.vi"("error in"=w292, "text"=w294) -> ()  [unwired: 9 in, 1 out]
      }
      frame "Confirm Quit" {
        # "Confirm Quit - Message that can confirm whether or not the user wants to exit the application."
        n120 = case shown="\"Acquiring and Logging\"" w318 {
          tunnel: w317 -> [w328 w335]
          tunnel: w316 -> [w327 w333]
          tunnel: [w321 w332] -> w314
          tunnel: [UI_State."Idle" ("UI State") w331] -> w315
          tunnel: w313 -> [w320 w330]
          frame Default {
            # "If 'Confirm Quit' comes in while the system is idle, there is no need for a confirmation message."
            n121 = call-poly "Enqueue Message.vi"("Priority Message? (F)"=TRUE, "error in (no error)"=w327, "Message"="Exit", "Message Queue"=w328) -> ("error out"=w321:errorcluster)  [unwired: 6 in, 1 out]
            n122 = Unbundle By Name(w320) -> ("TCU Module Config.Process Name"=w324:string)
            n123 = Concatenate Strings(w324, " Quit" ("text")) -> (w323:string)
            n124 = call "Write to Log File.vi"("error in"=w321, "text"=w323) -> ()  [unwired: 9 in, 1 out]
          }
          frame "Acquiring and Logging" {
            n125 = Two Button Dialog(message="Are you sure you want to quit while the acquisition is running?" ("Confirm Quit Message"), 1:"No" ("No"), 2:"Yes" ("Yes")) -> (T button?=w334:bool)
            n126 = case shown="True" w334 {
              tunnel: w335 -> [_ w349]
              tunnel: w333 -> [w339 w348]
              tunnel: [w339 w342] -> w332
              tunnel: [UI_State."Acquiring and Logging" ("UI State") UI_State."Waiting for Exit" ("UI State")] -> w331
              tunnel: w330 -> [_ w341]
              frame False {
                # "User did not want to quit."
              }
              frame True {
                n127 = call-poly "Enqueue Message.vi"("error in (no error)"=w348, "Message"="Stop", "Message Queue"=w349) -> ("error out"=w342:errorcluster)  [unwired: 7 in, 1 out]
                n128 = Unbundle By Name(w341) -> ("TCU Module Config.Process Name"=w345:string)
                n129 = Concatenate Strings(w345, " Quit" ("text")) -> (w344:string)
                n130 = call "Write to Log File.vi"("error in"=w342, "text"=w344) -> ()  [unwired: 9 in, 1 out]
              }
            }
          }
        }
      }
      frame "Display Log File Path" {
        n131 = Variant To Data(error in=w352, type=path "", Variant=w355) -> (data=→"Log File path":path, error out=w353:errorcluster)
      }
      frame "E-Stop" {
        # "Pause the TCU when E-Stop is pressed"
        # "Message Acquisition and Logging loops to stop"
        # "Enable: Start, Exit, Settings\nDisable: Stop"
        # "Stop the pumps."
        n132 = Unbundle By Name(w383) -> ("Trigger Ref"=w374:refnum<vi>, "Stop Ref"=w375:refnum<vi>, "Start Ref"=w378:refnum<vi>, "Exit Ref"=w377:refnum<vi>, "Settings Ref"=w376:refnum<vi>)
        n133 = call-poly "Enqueue Message.vi"("error in (no error)"=w367, "Message Data"="Ready..." ("Ready..."), "Message"="Update Status", "Message Queue"=w386) -> ("error out"=w369:errorcluster)  [unwired: 6 in, 1 out]
        n134 = Build Array(w378, w377, w376) -> (w381:refnum<vi>[])
        n135 = Build Array(w374, w375) -> (w380:refnum<vi>[])
        n136 = call-poly "Enqueue Message.vi"("error in (no error)"=w369, "Message"="Pause", "Message Queue"=w371) -> ("error out"=w368:errorcluster)  [unwired: 7 in, 1 out]
        n137 = call "Set Enable State on Multiple Controls.vi"("Enable?"=FALSE, "Controls"=w380) -> ()  [unwired: 10 in]
        n138 = call "Set Enable State on Multiple Controls.vi"("Enable?"=TRUE, "Controls"=w381) -> ()  [unwired: 10 in]
        n139 = case shown="Default" w372 {
          selector: w372 -> [_ w388]
          tunnel: [UI_State."Waiting for Stop" ("UI State") w388] -> w373
          frame Default {
          }
          frame "Waiting for Exit" {
          }
        }
        n140 = Bundle By Name(cluster=w365, "State"=State_Enum."Idle") -> (w362:T12)
        n141 = Merge Errors(w368) -> (w359:errorcluster)
        n142 = Unbundle By Name(w362) -> ("TCU Module Config.Process Name"=w360:string)
        n143 = call "Generate Temporary Report.vi"("error in (no error)"=w359, "Line of Events"=string[] ["E-STOP"], "Module Name"=w360) -> ("error out"=w358:errorcluster)  [unwired: 8 in]
        n144 = Concatenate Strings(w360, " E-STOP" ("text")) -> (w364:string)
        n145 = call "Write to Log File.vi"("error in"=w358, "text"=w364) -> ()  [unwired: 9 in, 1 out]
      }
      frame "Error" {
        # "Error - Check the error message data and respond accordingly. This message is sent by the \"Error Handler\" VIs at the end of each loop in this application."
        n146 = Variant To Data(error in=w404, type=errorcluster {"status"=FALSE, "code"=0, "source"=""} ("error out"), Variant=w403) -> (data=w401:errorcluster, error out=w397:errorcluster)
        n147 = call <vilib>:"General Error Handler.vi"("error in (no error)"=w401) -> ("message"=w389:string)  [unwired: 10 in, 4 out]
        n148 = call-poly "Enqueue Message.vi"("Priority Message? (F)"=TRUE, "Message"="Exit", "Message Queue"=w400) -> ("error out"=w396:errorcluster)  [unwired: 7 in, 1 out]
        n149 = Merge Errors(w396, w397) -> (w391:errorcluster)
        n150 = Unbundle By Name(w390) -> ("TCU Module Config.Process Name"=w394:string)
        n151 = Concatenate Strings(w394, " Error: " ("text"), w389) -> (w393:string)
        n152 = call "Write to Log File.vi"("error in"=w391, "text"=w393) -> ()  [unwired: 9 in, 1 out]
      }
      frame "Exit" {
        w417 = TRUE  # Delete Module?
        # "Don't check the error outs. The acquisition and logging queues may have already been released."
        # "Close references owned by the Main VI."
        # "Stop the VI"
        # "Exit - Fire the User Event to stop the Event Handling Loop.  Also send Exit messages to the Acquisition and Logging loops."
        n153 = Release Queue(queue=w427, error in (no error)=w431) -> (error out=w425:errorcluster)  [unwired: 1 in, 2 out]
        n154 = call "Fire User Event - Stop.vi"("User Event - Stop"=w430) -> ("error out"=w429:errorcluster)  [unwired: 10 in]
        n155 = Release Notifier(notifier=w426, error in (no error)=w425) -> (error out=w424:errorcluster)  [unwired: 1 in, 2 out]
        n156 = Build Array(w420) -> (w419:refnum<queue>[])
        n157 = Release Queue(queue=w422, error in (no error)=w424) -> (error out=w423:errorcluster)  [unwired: 1 in, 2 out]
        n158 = for {
          tunnel: w419 -> [w438] mode=indexing
          n159 = call-poly "Enqueue Message.vi"("Message"="Stop", "Message Queue"=w438) -> ("dup Message Queue"=w439:refnum<queue>)  [unwired: 8 in, 1 out]
          n160 = call-poly "Enqueue Message.vi"("Message"="Exit", "Message Queue"=w439) -> ()  [unwired: 8 in, 2 out]
        }
        n161 = Variant To Data(type=w417, Variant=w413) -> (data=w416:bool, error out=w418:errorcluster)  [unwired: 1 in]
        n162 = Select(t=w417, s=w418, f=w416) -> (s? t:f=w415:bool)
        n163 = case "Don't enqueue Delete Module if opening campaign because it\nwill already have been deleted and new config loaded and we create\na race condition." shown="True" w415 {
          tunnel: w414 -> [_ w435]
          tunnel: w410 -> [_ w434]
          frame False {
          }
          frame True {
            n164 = Unbundle By Name(w434) -> ("TCU Module Config.GUID"=w433:string)
            n165 = call-poly "Enqueue Message.vi"("Message Data"=w433, "Message"="Delete Module", "Message Queue"=w435) -> ()  [unwired: 7 in, 2 out]
          }
        }
        n166 = Merge Errors(w429, w423) -> (w407:errorcluster)
        n167 = Unbundle By Name(w410) -> ("TCU Module Config.Process Name"=w408:string)
        n168 = call "Generate Temporary Report.vi"("error in (no error)"=w407, "Line of Events"=string[] ["Exited"], "Module Name"=w408) -> ("error out"=w406:errorcluster)  [unwired: 8 in]
        n169 = Concatenate Strings(w408, " Exit" ("text")) -> (w412:string)
        n170 = call "Write to Log File.vi"("error in"=w406, "text"=w412) -> ()  [unwired: 9 in, 1 out]
      }
      frame "Init UI Refs" {
        # "Enable: Start, Exit, Settings\nDisable: Stop"
        # "Init UI Refs - Store control references for UI controls.  Also enable/disable controls appropriately."
        n171 = property class="VI"("Front Panel.Closeable"=TRUE ("Front Panel Window:Closeable")) -> ()  [unwired: 2 in, 2 out]
        n172 = control-ref of="Status"() -> (w446:refnum<vi>)
        n173 = control-ref of="Exit"() -> (w443:refnum<vi>)
        n174 = Bundle By Name(cluster=w449, "Status Ref"=w446, "Exit Ref"=w443) -> (w448:T4)
        n175 = Build Array(w443) -> (w445:refnum<vi>[])
        n176 = call "Set Enable State on Multiple Controls.vi"("Enable?"=TRUE, "Controls"=w445) -> ()  [unwired: 10 in]
      }
      frame "Initialize" {
        # "Initialize - Get configuration settings, then message the UI to initialize, and broadcast the settings to the other message loops."
        n177 = property class="VI" props=["FP.State"]() -> (reference out=w461:refnum<vi>)  [unwired: 2 in, 2 out]
        n178 = call-poly "Enqueue Message.vi"("error in (no error)"=w462, "Message"="Init UI Refs", "Message Queue"=w467) -> ("error out"=w465:errorcluster, "dup Message Queue"=w466:refnum<queue>)  [unwired: 7 in]
        n179 = call "Make Child and Move.vi"("Process Name"=w458, "Name of Parent Panel"=w459, "New Center Coords"=w460, "VI in"=w461) -> ()  [unwired: 8 in]
        n180 = call-poly "Enqueue Message.vi"("error in (no error)"=w465, "Message"="Broadcast Settings", "Message Queue"=w466) -> ("error out"=w473:errorcluster, "dup Message Queue"=w472:refnum<queue>)  [unwired: 7 in]
        n181 = call-poly "Enqueue Message.vi"("error in (no error)"=w473, "Message Data"="Ready..." ("Ready..."), "Message"="Update Status", "Message Queue"=w472) -> ("error out"=w452:errorcluster)  [unwired: 6 in, 1 out]
        n182 = Unbundle By Name(w455) -> ("TCU Module Config.Process Name"=w453:string)
        n183 = call "Generate Temporary Report.vi"("error in (no error)"=w452, "Line of Events"=string[] ["Initialized"], "Module Name"=w453) -> ("error out"=w451:errorcluster)  [unwired: 8 in]
        n184 = Concatenate Strings(w453, " Initialize" ("text")) -> (w457:string)
        n185 = call "Write to Log File.vi"("error in"=w451, "text"=w457) -> ()  [unwired: 9 in, 1 out]
      }
      frame "Launch Settings Dialog" {
        # "Launch the Settings Dialog when the user clicks the 'Settings' button."
        n186 = local read "TCU On?"() -> (w477:bool)
        n187 = in-place {
          in-place-border: w477 -> [w502]
          # "Keep track of the # of times the window is opened"
          n188 = in-place-cluster #3(w476) -> ("TCU Module Config.Load Count"=w504:i32)  [unwired: 1 out]
          n189 = Increment(x=w504) -> (x+1=w503:i32)
          n190 = in-place-cluster #3("TCU Module Config.Load Count"=w503, "TCU On?"=w502) -> (w475:T12)
        }
        n191 = call "TCU Settings Dialog.vi"("error in (no error)"=w485, "Message Queues"=w483, "TCU Module State Cluster In"=w475) -> ("error out"=w484:errorcluster, "Cancelled?"=w474:bool, "TCU Module Config Out"=w486:T5)  [unwired: 5 in, 1 out]
        n192 = disable-structure shown="Enabled" {
          disable-tunnel: w488 -> [w495 _]
          disable-tunnel: w487 -> [w494 _]
          disable-tunnel: w484 -> [w493 w501]
          disable-tunnel: [w492 w501] -> w479
          disable-tunnel: w474 -> [w491 _]
          frame Disabled {
            n193 = case shown="False" w491 {
              tunnel: w493 -> [w499 w500]
              tunnel: [w497 w500] -> w492
              tunnel: w495 -> [_ _]
              tunnel: w494 -> [w498 _]
              frame False {
                n194 = call-poly "Enqueue Message.vi"("error in (no error)"=w499, "Message"="Broadcast Settings", "Message Queue"=w498) -> ("error out"=w497:errorcluster)  [unwired: 7 in, 1 out]
              }
              frame True {
              }
            }
          }
          frame Enabled {
          }
        }
        n195 = Bundle By Name(cluster=w476, "TCU Module Config"=w486) -> (w478:T12)
        n196 = Unbundle By Name(w478) -> ("TCU Module Config.Process Name"=w482:string)
        n197 = Concatenate Strings(w482, " Settings Dialog Launched" ("text")) -> (w481:string)
        n198 = call "Write to Log File.vi"("error in"=w479, "text"=w481) -> ()  [unwired: 9 in, 1 out]
      }
      frame "Logging Stopped" {
        # "Logic for determining what action to take when the logging has stopped."
        n199 = case shown="\"Waiting for Exit (Acq Stopped)\"" w513 {
          selector: w513 -> [w516 _ _ _ _]
          tunnel: [w516 UI_State."Waiting for Exit (Log Stopped)" ("UI State") UI_State."Waiting for Stop (Log Stopped)" ("UI State") UI_State."Idle" ("UI State") UI_State."Idle" ("UI State")] -> w512
          tunnel: w511 -> [w515 w517 w519 w525 w531]
          tunnel: [w515 w517 w519 w524 w530] -> w506
          tunnel: w510 -> [_ _ _ w523 w529]
          frame Default {
          }
          frame "Waiting for Exit", "Waiting for Exit (Log Stopped)" {
          }
          frame "Waiting for Stop", "Waiting for Stop (Log Stopped)" {
          }
          frame "Waiting for Exit (Acq Stopped)" {
            # "If we are waiting to exit, and the acquisition has already stopped, then the \"Logging Stopped\" message indicates that it is time to exit."
            n200 = call-poly "Enqueue Message.vi"("Priority Message? (F)"=TRUE, "error in (no error)"=w525, "Message"="Exit", "Message Queue"=w523) -> ("error out"=w524:errorcluster)  [unwired: 6 in, 1 out]
          }
          frame "Waiting for Stop (Acq Stopped)" {
            # "If we are waiting to stop, and the acquisition has already stopped, then the \"Logging Stopped\" message indicates that it is time to stop."
            n201 = call-poly "Enqueue Message.vi"("error in (no error)"=w531, "Message Data"="Ready..." ("Message"), "Message"="Update Status", "Message Queue"=w529) -> ("error out"=w530:errorcluster)  [unwired: 6 in, 1 out]
          }
        }
        n202 = Unbundle By Name(w505) -> ("TCU Module Config.Process Name"=w509:string)
        n203 = Concatenate Strings(w509, " Logging Stopped" ("text")) -> (w508:string)
        n204 = call "Write to Log File.vi"("error in"=w506, "text"=w508) -> ()  [unwired: 9 in, 1 out]
      }
      frame "Send to Sequence" {
        n205 = Variant To Data(error in=w538, type=refnum<queue> refnum ("Message Queue"), Variant=w535) -> (data=w536:refnum<queue>, error out=w537:errorcluster)
        n206 = local read "Display Cluster"() -> (w534:cluster{"User Name":string, "Temp Display":dbl})
        n207 = Unbundle By Name(w534) -> ("Temp Display"=w533:dbl)
        n208 = call-poly "Enqueue Message.vi"("error in (no error)"=w537, "Message Data"=w533, "Message"="Sent to Sequence", "Message Queue"=w536) -> ("error out"=w542:errorcluster)  [unwired: 6 in, 1 out]
      }
      frame "Start" {
        # "Clear chart"
        # "Message Acquisition and Logging loops to start"
        # "Enable: Stop\nDisable: Start, Exit, Settings"
        # "Start - Enable/Disable buttons appropriately for an acquisition that has started, and update status display."
        n209 = Unbundle By Name(w552) -> ("Trigger Ref"=w563:refnum<vi>, "Stop Ref"=w564:refnum<vi>, "Start Ref"=w567:refnum<vi>, "Exit Ref"=w566:refnum<vi>, "Settings Ref"=w565:refnum<vi>, "Data Ref"=w554:refnum<vi>)
        n210 = property class="WFChart (strict)"(reference=w554, "History Data"=waveform(dbl)[][] []) -> ()  [unwired: 1 in, 2 out]
        n211 = Build Array(w567, w566, w565) -> (w570:refnum<vi>[])
        n212 = Build Array(w563, w564) -> (w569:refnum<vi>[])
        n213 = call-poly "Enqueue Message.vi"("error in (no error)"=w555, "Message"="Broadcast settings", "Message Queue"=w557) -> ("error out"=w558:errorcluster, "dup Message Queue"=w556:refnum<queue>)  [unwired: 7 in]
        n214 = call "Set Enable State on Multiple Controls.vi"("Enable?"=TRUE, "Controls"=w569) -> ()  [unwired: 10 in]
        n215 = call "Set Enable State on Multiple Controls.vi"("Enable?"=FALSE, "Controls"=w570) -> ()  [unwired: 10 in]
        n216 = call-poly "Enqueue Message.vi"("error in (no error)"=w558, "Message"="Start Loops", "Message Queue"=w556) -> ("error out"=w559:errorcluster)  [unwired: 7 in, 1 out]
        n217 = Merge Errors(w559) -> (w546:errorcluster)
        n218 = Bundle By Name(cluster=w551, "State"=State_Enum."Measuring") -> (w545:T12)
        n219 = Unbundle By Name(w545) -> ("TCU Module Config.Process Name"=w549:string)
        n220 = Concatenate Strings(w549, " Start" ("text")) -> (w548:string)
        n221 = call "Write to Log File.vi"("error in"=w546, "text"=w548) -> ()  [unwired: 9 in, 1 out]
      }
      frame "Sequence Start" {
        # "Start the sequence if it is not already running"
        # "Clear chart"
        # "Message Acquisition and Logging loops to start"
        # "Enable: Stop\nDisable: Start, Exit, Settings"
        # "Start - Enable/Disable buttons appropriately for an acquisition that has started, and update status display."
        n222 = Unbundle By Name(w584) -> ("Trigger Ref"=w591:refnum<vi>, "Stop Ref"=w592:refnum<vi>, "Start Ref"=w595:refnum<vi>, "Exit Ref"=w594:refnum<vi>, "Settings Ref"=w593:refnum<vi>, "Data Ref"=w586:refnum<vi>)
        n223 = property class="WFChart (strict)"(reference=w586, "History Data"=waveform(dbl)[][] []) -> ()  [unwired: 1 in, 2 out]
        n224 = Build Array(w595, w594, w593) -> (w598:refnum<vi>[])
        n225 = Build Array(w591, w592) -> (w597:refnum<vi>[])
        n226 = call-poly "Enqueue Message.vi"("error in (no error)"=w587, "Message"="Broadcast settings", "Message Queue"=w588) -> ("error out"=w580:errorcluster, "dup Message Queue"=w581:refnum<queue>)  [unwired: 7 in]
        n227 = call "Set Enable State on Multiple Controls.vi"("Enable?"=TRUE, "Controls"=w597) -> ()  [unwired: 10 in]
        n228 = call "Set Enable State on Multiple Controls.vi"("Enable?"=FALSE, "Controls"=w598) -> ()  [unwired: 10 in]
        n229 = case shown="False" w578 {
          selector: w578 -> [_ w605]
          tunnel: [TRUE w605] -> w577
          tunnel: w580 -> [w603 w606]
          tunnel: w581 -> [w601 _]
          tunnel: [w600 w606] -> w579
          frame False {
            n230 = call-poly "Enqueue Message.vi"("error in (no error)"=w603, "Message"="Start Loops", "Message Queue"=w601) -> ("error out"=w600:errorcluster)  [unwired: 7 in, 1 out]
          }
          frame True {
          }
        }
        n231 = Merge Errors(w579) -> (w573:errorcluster)
        n232 = Bundle By Name(cluster=w583, "State"=State_Enum."Measuring") -> (w572:T12)
        n233 = Unbundle By Name(w572) -> ("TCU Module Config.Process Name"=w576:string)
        n234 = Concatenate Strings(w576, " Sequence Start" ("text")) -> (w575:string)
        n235 = call "Write to Log File.vi"("error in"=w573, "text"=w575) -> ()  [unwired: 9 in, 1 out]
      }
      frame "Start Loops" {
        # "We don't have multiple Process Names per module, but i am leaving it for now."
        # "Message Acquisition and Logging loops to start"
        # "Start - Enable/Disable buttons appropriately for an acquisition that has started, and update status display."
        n236 = Build Array(w615) -> (w613:refnum<queue>[])
        n237 = Unbundle By Name(w612) -> ("TCU Module Config.Process Name"=w609:string)
        n238 = for {
          tunnel: w611 -> [w621]
          tunnel: [w620] -> w614 mode=indexing
          tunnel: w613 -> [w619] mode=indexing
          tunnel: w609 -> [w618]
          n239 = call-poly "Enqueue Message.vi"("error in (no error)"=w621, "Message Data"=w618, "Message"="Start", "Message Queue"=w619) -> ("error out"=w620:errorcluster)  [unwired: 6 in, 1 out]
        }
        n240 = Merge Errors(w611, w614) -> (w608:errorcluster)
        n241 = call "Generate Temporary Report.vi"("error in (no error)"=w608, "Line of Events"=string[] ["Started"], "Module Name"=w609) -> ("error out"=w607:errorcluster)  [unwired: 8 in]
      }
      frame "Start Log" {
        # "Message Acquisition and Logging loops to start"
        # "Start - Enable/Disable buttons appropriately for an acquisition that has started, and update status display."
        n242 = Build Array(w632) -> (w630:refnum<queue>[])
        n243 = Unbundle By Name(w624) -> ("TCU Module Config.Process Name"=w629:string)
        n244 = for {
          tunnel: w623 -> [w638]
          tunnel: [w637] -> w631 mode=indexing
          tunnel: w630 -> [w636] mode=indexing
          tunnel: w629 -> [w635]
          n245 = call-poly "Enqueue Message.vi"("error in (no error)"=w638, "Message Data"=w635, "Message"="Start Log", "Message Queue"=w636) -> ("error out"=w637:errorcluster)  [unwired: 6 in, 1 out]
        }
        n246 = Merge Errors(w623, w631) -> (w625:errorcluster)
        n247 = Unbundle By Name(w624) -> ("TCU Module Config.Process Name"=w628:string)
        n248 = Concatenate Strings(w628, " Start Log" ("text")) -> (w627:string)
        n249 = call "Write to Log File.vi"("error in"=w625, "text"=w627) -> ()  [unwired: 9 in, 1 out]
      }
      frame "Stop" {
        # "Pause the TCU on Stop"
        # "Enable: Start, Exit, Settings\nDisable: Stop"
        # "Stop - Enable/Disable buttons appropriately for an acquisition that has stopped, and update status display."
        n250 = Unbundle By Name(w669) -> ("Trigger Ref"=w660:refnum<vi>, "Stop Ref"=w661:refnum<vi>, "Start Ref"=w664:refnum<vi>, "Exit Ref"=w663:refnum<vi>, "Settings Ref"=w662:refnum<vi>)
        n251 = call-poly "Enqueue Message.vi"("error in (no error)"=w645, "Message"="Broadcast settings", "Message Queue"=w647) -> ("error out"=w644:errorcluster, "dup Message Queue"=w646:refnum<queue>)  [unwired: 7 in]
        n252 = Build Array(w664, w663, w662) -> (w667:refnum<vi>[])
        n253 = Build Array(w660, w661) -> (w666:refnum<vi>[])
        n254 = call-poly "Enqueue Message.vi"("error in (no error)"=w644, "Message Data"="Ready..." ("Ready..."), "Message"="Update Status", "Message Queue"=w646) -> ("error out"=w656:errorcluster)  [unwired: 6 in, 1 out]
        n255 = call "Set Enable State on Multiple Controls.vi"("Enable?"=FALSE, "Controls"=w666) -> ()  [unwired: 10 in]
        n256 = call "Set Enable State on Multiple Controls.vi"("Enable?"=TRUE, "Controls"=w667) -> ()  [unwired: 10 in]
        n257 = call-poly "Enqueue Message.vi"("error in (no error)"=w656, "Message"="Pause", "Message Queue"=w657) -> ("error out"=w654:errorcluster)  [unwired: 7 in, 1 out]
        n258 = case shown="\"Waiting for Exit\"" w658 {
          selector: w658 -> [_ w673]
          tunnel: [UI_State."Waiting for Stop" ("UI State") w673] -> w659
          frame Default {
          }
          frame "Waiting for Exit" {
          }
        }
        n259 = Merge Errors(w654) -> (w641:errorcluster)
        n260 = Bundle By Name(cluster=w653, "State"=State_Enum."Paused") -> (w649:T12)
        n261 = Unbundle By Name(w649) -> ("TCU Module Config.Process Name"=w642:string)
        n262 = call "Generate Temporary Report.vi"("error in (no error)"=w641, "Line of Events"=string[] ["Stopped"], "Module Name"=w642) -> ("error out"=w640:errorcluster)  [unwired: 8 in]
        n263 = Concatenate Strings(w642, " Stop" ("text")) -> (w651:string)
        n264 = call "Write to Log File.vi"("error in"=w640, "text"=w651) -> ()  [unwired: 9 in, 1 out]
      }
      frame "Update Status" {
        # "Update Display - Convert the message data to a string to display in the Status indicator."
        n265 = Variant To Data(error in=w684, type="", Variant=w683) -> (data=w677:string, error out=w681:errorcluster)
        "Status" <- w677
        n266 = Unbundle By Name(w680) -> ("Trigger Ref"=w676:refnum<vi>, "Stop Ref"=w679:refnum<vi>)
        n267 = property class="Bool"(reference=w679) -> ("DisabledEnum"=w678:T20)  [unwired: 1 in, 2 out]
        n268 = case shown="\"Enabled\"" w678 {
          tunnel: w677 -> [w688 _]
          tunnel: w676 -> [w689 _]
          frame "Enabled" {
            # "Disable the Force Trigger only while we are logging."
            n269 = Build Array(w689) -> (w690:refnum<vi>[])
            n270 = Not Equal?(x="Logging" ("Logging"), y=w688) -> (x != y?=w686:bool)
            n271 = call "Set Enable State on Multiple Controls.vi"("Enable?"=w686, "Controls"=w690) -> ()  [unwired: 10 in]
          }
          frame "Disabled", Default {
          }
        }
        n272 = Merge Errors(w681) -> (w685:errorcluster)
      }
      frame Default {
        # "'Default' case only runs if there is a message that isn't defined in any of the other cases.  Output a programming error."
        n273 = Concatenate Strings("The invalid message string " ("string"), w692, " was received in TCU Main." ("string")) -> (w693:string)
        n274 = Bundle By Name(cluster=errorcluster {"status"=TRUE, "code"=1, "source"=""} ("error constant"), "source"=w693) -> (w691:errorcluster)
        n275 = Unbundle By Name(w697) -> ("TCU Module Config.Process Name"=w700:string)
        n276 = Concatenate Strings(w700, " Incorrect Message Recieved: " ("text"), w692) -> (w699:string)
        n277 = call "Write to Log File.vi"("error in"=w691, "text"=w699) -> ()  [unwired: 9 in, 1 out]
      }
    }
    n278 = call "Error Handler - Message Handling Loop.vi"("error in (no error)"=w159, "Message Queue"=w157) -> ("dup error in"=w158:errorcluster, "dup Message Queue"=w143:refnum<queue>)  [unwired: 8 in]
  }
  n279 = call "Main Loop.vi"("error in (no error)"=w9, "Chart Notifier"=w16, "Message Queues"=w10) -> ("error out"=w17:errorcluster)  [unwired: 8 in]
  n280 = Release Queue(queue=w4) -> ()  [unwired: 2 in, 3 out]
  n281 = Close Reference(reference=w15) -> ()  [unwired: 1 in, 1 out]
  n282 = Unregister For Events(event registration refnum=w23, error in=w28) -> (error out=w24:errorcluster)
  n283 = Release Queue(queue=w3) -> ()  [unwired: 2 in, 3 out]
  n284 = Merge Errors(w24, w29, w9, w17) -> (w27:errorcluster)
  n285 = Release Queue(queue=w2) -> ()  [unwired: 2 in, 3 out]
  n286 = call "Destroy User Event - Stop.vi"("error in (no error)"=w27, "User Event - Stop"=w25) -> ()  [unwired: 9 in, 1 out]
